vi "Write E and F Params.vi"(6 "Input Positive (E,F)":bool, 8 "error in (no error)":errorcluster, 9 "Onto MsBus (E,F)":bool, 10 "Disconnect (E,F)":bool, 11 "BME_DG_G08_Chnl in":refnum<class "BME_DG_G05P2_Chnl.lvclass">) -> (0 "error out":errorcluster, 3 "BME_DG_G08_Chnl out":refnum<class "BME_DG_G05P2_Chnl.lvclass">)   [LabVIEW 2009]
uses:
  BME_DG_G05P2_Chnl.lvclass
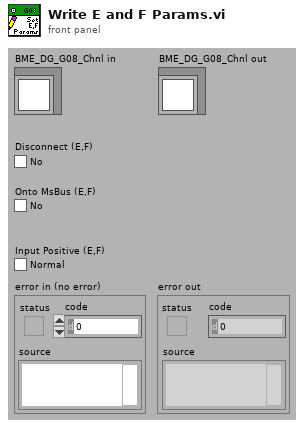
[diagram p1: front panel]
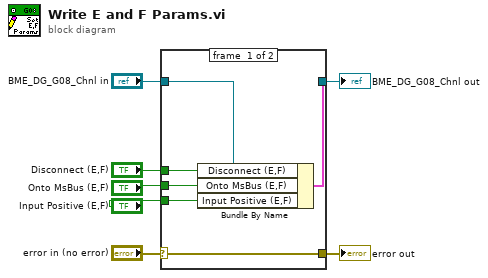
[diagram p0: block diagram]
diagram:
  n1 = case shown="No Error" "error in (no error)" {
    selector: "error in (no error)" -> [w13 w14]
    tunnel: [w13 w14] -> w6
    tunnel: [w11 w15] -> w4
    tunnel: "BME_DG_G08_Chnl in" -> [w12 w15]
    tunnel: "Disconnect (E,F)" -> [w10 _]
    tunnel: "Onto MsBus (E,F)" -> [w9 _]
    tunnel: "Input Positive (E,F)" -> [w8 _]
    frame #0 {
      n2 = Bundle By Name(cluster=w12, "Disconnect (E,F)"=w10, "Onto MsBus (E,F)"=w9, "Input Positive (E,F)"=w8) -> (w11:cluster{})
    }
    frame #1 {
    }
  }
  "error out" <- w6
  "BME_DG_G08_Chnl out" <- w4
